vi "V7310.Start.vi"(6 "timeout ms (5000)":i32=5000, 8 "error in":errorcluster, 11 "Connection in":refnum<k5>) -> (0 "error out":errorcluster, 3 "Connection out":refnum<k5>)   [LabVIEW 2016]
uses:
  LowLevel/V7310.Commands.ctl
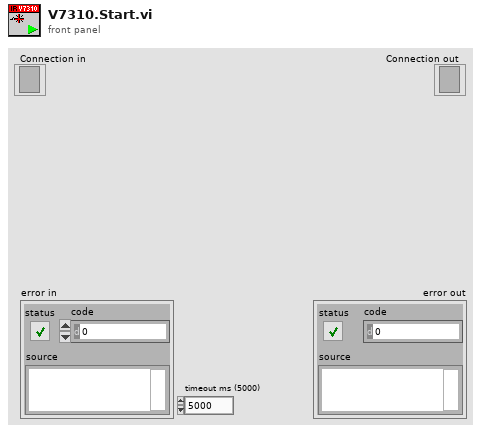
[diagram p1: front panel]
types:
  T1 = typedef "V7310.Commands.ctl" = enum16{"Start", "Stop", "GetStatus", "GetVarNames", "GetJobNames", "SetJob", "GetJob", "SetVars", "GetVars", "SetLayoutPosition", "SetRotation", "GetMessageID", "GetMessages", "ConfirmMessages", "DeleteMessages", "SetRTC", "GetRTC", "SetVarPosition", "SetIntensity", "GetIntensity", "SetStartTriggerDelay", "GetStartTriggerDelay", "SetStopTriggerDelay", "GetStopTriggerDelay", "SetConsecutiveTriggerDelay", "GetConsecutiveTriggerDelay", "SetMarkSpeed", "GetMarkSpeed"}
  T2 = typedef "V7310.ErrorLevels.ctl" = enum16{"OK", "Warning", "Error"}
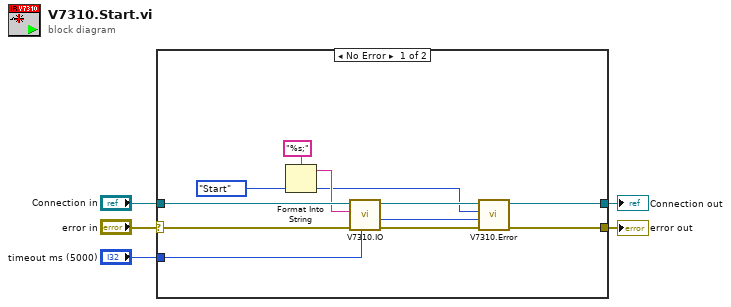
[diagram p0: block diagram]
diagram:
  n1 = case shown="No Error" "error in" {
    selector: "error in" -> [w13 w16]
    tunnel: "Connection in" -> [w14 w17]
    tunnel: [w15 w17] -> w4
    tunnel: "timeout ms (5000)" -> [w12 _]
    tunnel: [w6 w16] -> w1
    frame No Error {
      w9 = V7310.Commands."Start" ("Cmd")
      n2 = Format Into String(format string="%s;", w9) -> (resulting string=w10:string)  [unwired: 2 in, 1 out]
      n3 = call "V7310.IO.vi"("timeout ms (5000)"=w12, "error in"=w13, "Data in"=w10, "Connection in"=w14) -> ("error out"=w7:errorcluster, "Error Level"=w8:T2, "Connection out"=w15:refnum<k5>)  [unwired: 4 in, 1 out]
      n4 = call "V7310.Error.vi"("error in"=w7, "Error Level"=w8, "Cmd"=w9) -> ("error out"=w6:errorcluster)  [unwired: 8 in]
    }
    frame Error {
    }
  }
  "Connection out" <- w4
  "error out" <- w1
